vi "Flatten.vi"(8 "error in (no error)":errorcluster, 11 "Wavelength iHR320 in":refnum<class "Wavelength ActiveX.lvclass">) -> (0 "error out":errorcluster, 3 "Wavelength iHR320 out":refnum<class "Wavelength ActiveX.lvclass">)   [LabVIEW 2015, in "Wavelength ActiveX.lvclass"]
uses:
  Wavelength ActiveX.lvclass
  Wavelength ActiveX.lvclass/Wavelength ActiveX.ctl
  Global/File Locations.vi
  Scanner/Scanner.lvclass
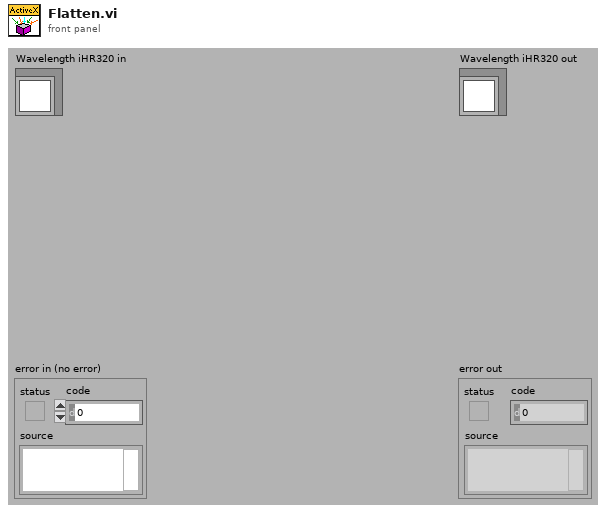
[diagram p1: front panel]
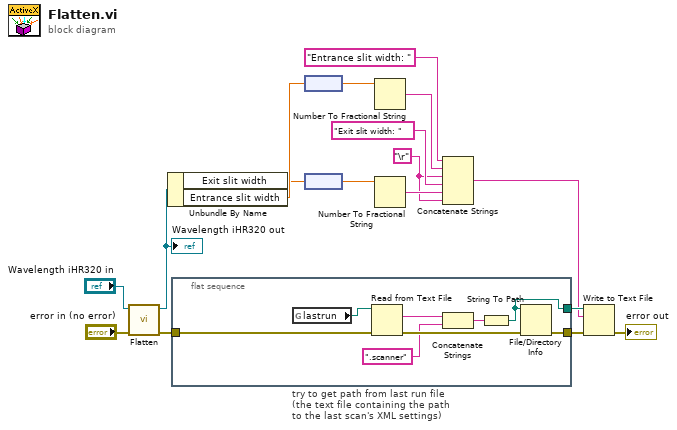
[diagram p0: block diagram]
diagram:
  w2 = "\r"
  n1 = call-parent "Flatten.vi"("error in (no error)"="error in (no error)", "Scanner in"="Wavelength iHR320 in") -> ("error out"=w15:errorcluster, "Scanner out"=w11:refnum<class "Wavelength ActiveX.lvclass">)  [unwired: 8 in]
  "Wavelength iHR320 out" <- w11
  n2 = Unbundle By Name(w11) -> ("Exit slit width"=w8:dbl[unit], "Entrance slit width"=w10:dbl[unit])
  n3 = flat-sequence "try to get path from last run file\n(the text file containing the path\nto the last scan's XML settings)" {
    tunnel: [w25] -> w12
    tunnel: [w22] -> w13
    tunnel: w15 -> [w21]
    frame #0 {
      n4 = global read "File Locations.vi" "lastrun"() -> (w24:path)
      n5 = Read from Text File(file (use dialog)=w24, error in=w21) -> (text=w20:string, error out=w23:errorcluster)  [unwired: 4 out]
      n6 = Concatenate Strings(w20, ".scanner") -> (w18:string)
      n7 = String To Path(string=w18) -> (path=w25:path)
      n8 = File/Directory Info(path=w25, error in=w23) -> (error out=w22:errorcluster)  [unwired: 6 out]
    }
  }
  n9 = node(w10) -> (w9:dbl)
  n10 = node(w8) -> (w7:dbl)
  n11 = Number To Fractional String(number=w9) -> (F-format string=w4:string)  [unwired: 3 in]
  n12 = Number To Fractional String(number=w7) -> (F-format string=w3:string)  [unwired: 3 in]
  n13 = Concatenate Strings("Entrance slit width: ", w4, w2, "Exit slit width: ", w3, w2) -> (w1:string)
  n14 = Write to Text File(file (use dialog)=w12, text=w1, error in=w13) -> (error out=→"error out":errorcluster)  [unwired: 1 in, 2 out]
